vi "_Update Service Info.vi"(8 "error in (no error)":errorcluster, 10 "Service":T1, 11 "DiscoveryService in":refnum<class "NodeDiscovery.lvclass">) -> (0 "error out":errorcluster, 3 "DiscoveryService out":refnum<class "NodeDiscovery.lvclass">)   [LabVIEW 2020, in "Vecto.lvlib" / "NodeDiscovery.lvclass"]
uses:
  NodeDiscovery.lvclass
  proto/Service/Data.ctl
  proto/ServiceType/Enumeration.ctl
  NodeDiscovery.lvclass/NodeDiscovery.ctl
  proto/Discovery/Class/Msg.lvclass/Msg.ctl
  proto/Discovery/Class/Msg.lvclass
  proto/ServiceType/ServiceType.lvlib
  proto/Service/Service.lvlib
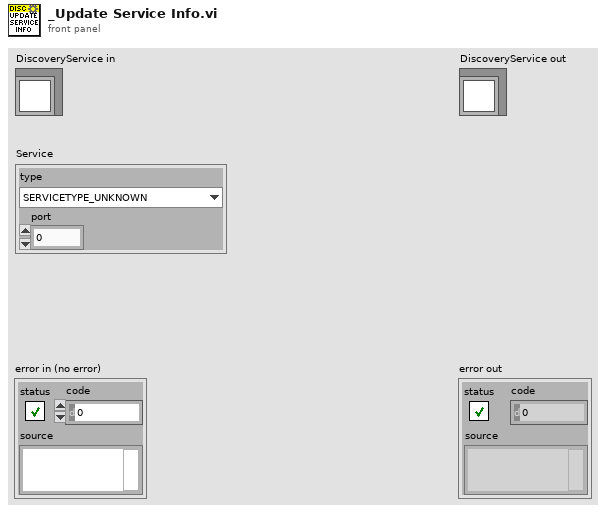
[diagram p1: front panel]
types:
  T1 = typedef "Service.lvlib/Data.ctl" = cluster{"type":T2, "port":i32}
  T2 = typedef "ServiceType.lvlib/Enumeration.ctl" = enum16{"SERVICETYPE_UNKNOWN", "SERVICETYPE_TCPSERVER", "SERVICETYPE_HTTPSERVER"}
  T3 = typedef "Discovery.lvlib/Data.ctl" = cluster{"node_id":u32, "name":string, "ip":u32, "status":string, "services":T1[], "system":string, "cluster":string}
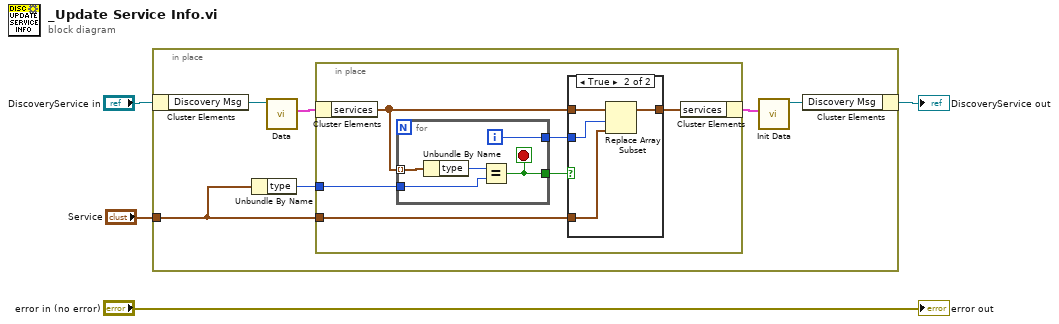
[diagram p0: block diagram]
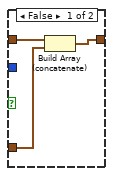
[diagram p2: hidden frame]
diagram:
  n1 = in-place {
    in-place-border: "Service" -> [w7]
    n2 = in-place-cluster #1("DiscoveryService in") -> ("Discovery Msg"=w10:refnum<class "Msg.lvclass">)
    n3 = Unbundle By Name(w7) -> ("type"=w8:T2)
    n4 = call "Data.vi"("PB Msg Template in"=w10) -> ("Data"=w9:T3)  [unwired: 8 in, 2 out]
    n5 = in-place {
      in-place-border: w8 -> [w16]
      in-place-border: w7 -> [w11]
      n6 = in-place-cluster #2(w9) -> ("services"=w13:T1[])
      n7 = for {
        tunnel: w13 -> [w28] mode=indexing
        tunnel: w16 -> [w27]
        tunnel: [w25] -> w14
        tunnel: [w24] -> w15
        i -> [w25]
        stop <- w24 stop-if-true
        n8 = Unbundle By Name(w28) -> ("type"=w26:T2)
        n9 = Equal?(x=w26, y=w27) -> (x = y?=w24:bool)
      }
      n10 = case shown="True" w15 {
        tunnel: w14 -> [_ w20]
        tunnel: w13 -> [w19 w23]
        tunnel: [w17 w22] -> w12
        tunnel: w11 -> [w18 w21]
        frame False {
          n11 = Build Array (concatenate)(w19, w18) -> (w17:T1[])
        }
        frame True {
          n12 = Replace Array Subset(array=w23, new element=w21, index=w20) -> (w22:T1[])
        }
      }
      n13 = in-place-cluster #2("services"=w12) -> (w6:T3)
    }
    n14 = call "Init Data.vi"("Data"=w6) -> ("Msg out"=w5:refnum<class "Msg.lvclass">)  [unwired: 10 in]
    n15 = in-place-cluster #1("Discovery Msg"=w5) -> (→"DiscoveryService out":refnum<class "NodeDiscovery.lvclass">)
  }
  "error out" <- "error in (no error)"
